vi "Post Build Script (auto build).vi"(8 "Package Source Folder":path=path "C:/user/patrick/git/Multichannel-Lockin/src", 9 "Package Version":string="2.8.9.18", 10 "Product Name":string="Multichannel Lockin", 11 "Output Package File Path":path) -> (0 "error out":errorcluster)   [LabVIEW 2016, in "PostBuildSupport.lvclass"]
uses:
  PostBuildSupport.lvclass
  PostBuildSupport.lvclass/PostBuildSupport.ctl
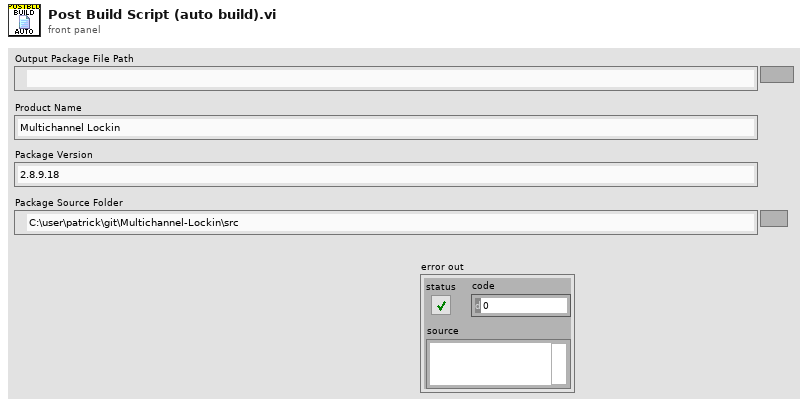
[diagram p1: front panel]
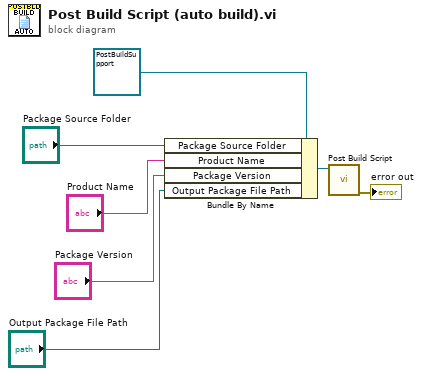
[diagram p0: block diagram]
diagram:
  n1 = Bundle By Name(cluster=refnum<class "PostBuildSupport.lvclass"> refnum ("PostBuildSupport in"), "Package Source Folder"="Package Source Folder", "Product Name"="Product Name", "Package Version"="Package Version", "Output Package File Path"="Output Package File Path") -> (w2:refnum<class "PostBuildSupport.lvclass">)
  n2 = call "Post Build Script.vi"("PostBuildSupport in"=w2) -> ("error out"=→"error out":errorcluster)  [unwired: 10 in]
